vi "Set Property.vi"(5 "property value":variant, 7 "property name":string, 8 "error in (no error)":errorcluster, 9 "channel name":string, 10 "group name":string, 11 "Logger in":refnum<class "Logger.lvclass">) -> (0 "error out":errorcluster, 1 "channel name out":string, 2 "group name out":string, 3 "Logger out":refnum<class "Logger.lvclass">)   [LabVIEW 2016, in "Logger.lvclass"]
uses:
  Logger.lvclass
  Logger.lvclass/Logger.ctl
  Read File.lvclass.vi
  Write File.lvclass.vi
  NHMFL_Core/Libraries/File/File Class/File.lvclass
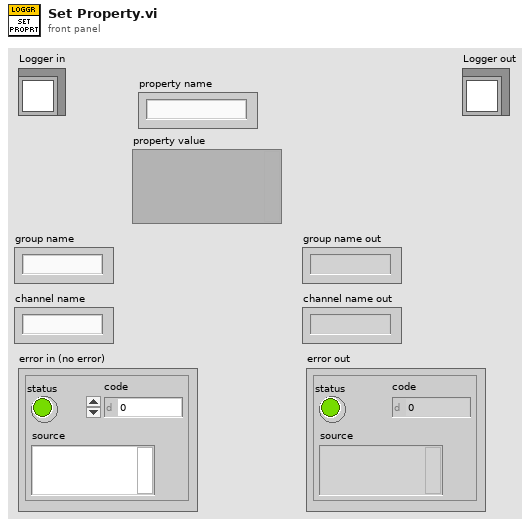
[diagram p1: front panel]
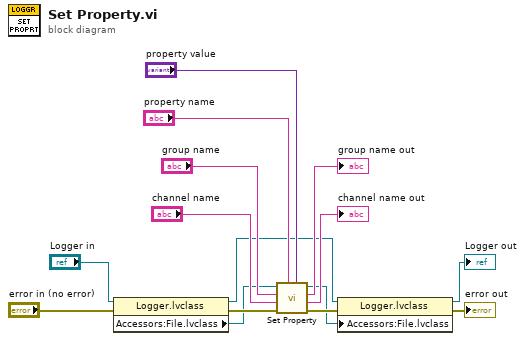
[diagram p0: block diagram]
diagram:
  n1 = property class="Logger.lvclass"(reference="Logger in", error in="error in (no error)") -> (reference out=w4:refnum<class "Logger.lvclass">, error out=w7:errorcluster, "Accessors:File.lvclass"=w2:refnum<class "File.lvclass">)
  n2 = call-dynamic "Set Property.vi"("property value"="property value", "property name"="property name", "error in (no error)"=w7, "channel name"="channel name", "group name"="group name", "File in"=w2) -> ("error out"=w8:errorcluster, "channel name out"=→"channel name out":string, "group name out"=→"group name out":string, "File out"=w1:refnum<class "File.lvclass">)  [unwired: 2 in]
  n3 = property class="Logger.lvclass"(reference=w4, error in=w8, "Accessors:File.lvclass"=w1) -> (reference out=→"Logger out":refnum<class "Logger.lvclass">, error out=→"error out":errorcluster)
